vi "Mapping Countdown v10.5.1.vi"(6 "Execution Times (s)":dbl[](array[numeric]), 8 "Drive Velocity":dbl=10.0 caption="Velocity (V/s)" min=10.0 max=160.0 step=0.1 format="%.1f", 9 "Mapping Spectra Settings":T1={"Integration Time"=10.0, "Repetitions"=10, "Mapping Spectra"=TRUE} {"Repetitions" min=1 max=100 step=1; "Integration Time" min=0.5 max=6000.0 step=1.0 format="%.1f"}, 10 "Ready Steps":i32, 11 "Mapping Drive Parameters":T2={"X Start Position"=10.0, "X Stop Position"=10.0, "Y Start Position"=10.0, "Y Stop Position"=10.0, "Step Size"=10.0} {"Step Size" min=0.1 max=30.0 step=0.1 format="%.1f"; "Y Stop Position" min=0.0 max=30.0 step=0.1 format="%.1f"; "Y Start Position" min=0.0 max=30.0 step=0.1 format="%.1f"; "X Stop Position" min=0.0 max=30.0 step=0.1 format="%.1f"; "X Start Position" min=0.0 max=30.0 step=0.1 format="%.1f"}) -> (2 "Progress":i16, 3 "Time String":string)   [LabVIEW 2010]
uses:
  TypeDefs/Mapping Drive Params.ctl
  TypeDefs/Mapping Spectra Params.ctl
  <vilib>/Analysis/NI_AALBase.lvlib
panel:
  out "Step Time (s)":dbl
  out "Left Time (s)":dbl
  out "Left Steps":dbl
  out "Total Steps":dbl
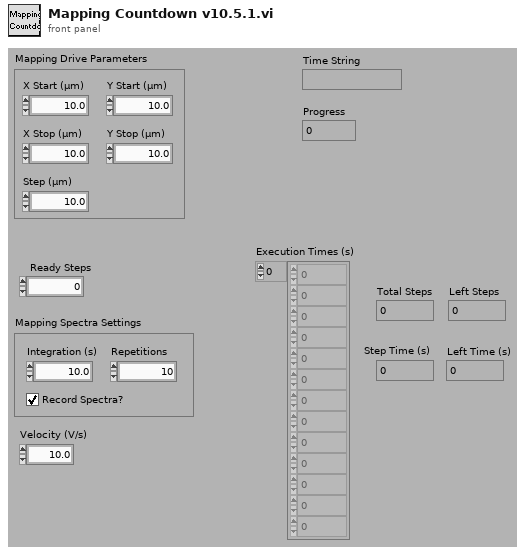
[diagram p1: front panel]
types:
  T1 = typedef "Mapping Spectra Params.ctl" = cluster{"Integration Time":dbl, "Repetitions":u16, "Mapping Spectra":bool}
  T2 = typedef "Mapping Drive Params.ctl" = cluster{"X Start Position":dbl, "X Stop Position":dbl, "Y Start Position":dbl, "Y Stop Position":dbl, "Step Size":dbl}
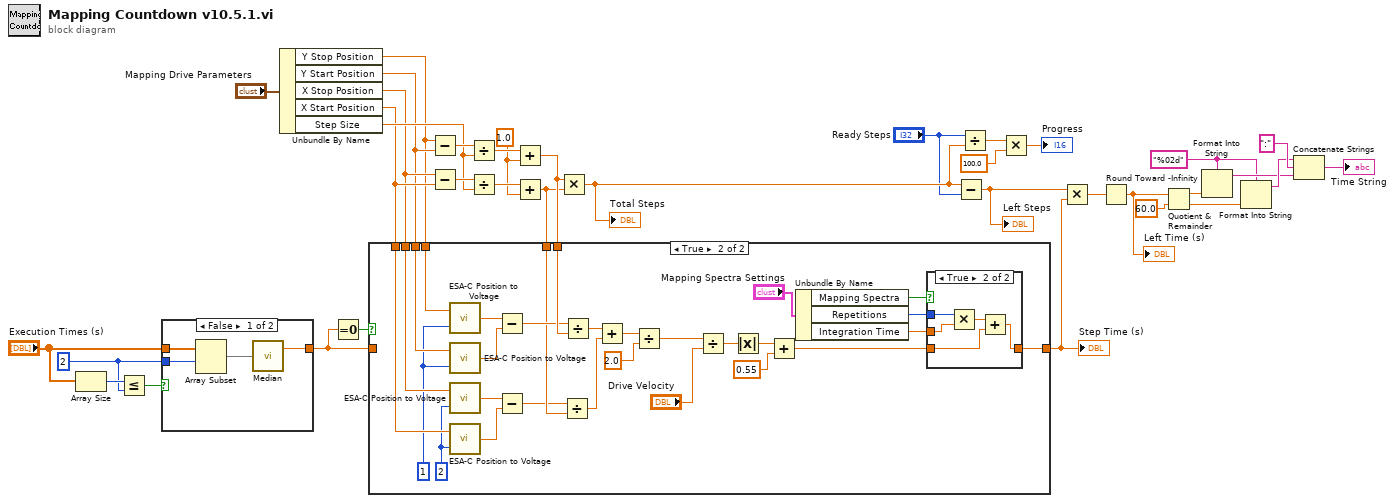
[diagram p0: block diagram]
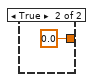
[diagram p2: hidden frame]
diagram:
  w4 = 2 ("index")
  w19 = 1.0 ("y")
  w31 = "%02d" ("Format-String")
  n1 = Array Size(array="Execution Times (s)") -> (size(s)=w7:i32)
  n2 = Less Or Equal?(x=w7, y=w4) -> (x <= y?=w6:bool)
  n3 = case shown="False" w6 {
    tunnel: "Execution Times (s)" -> [w39 _]
    tunnel: w4 -> [w38 _]
    tunnel: [w37 0.0 ("mean")] -> w3
    frame False {
      n4 = Array Subset(array=w39, index=w38) -> (w40:dbl[])  [unwired: 1 in]
      n5 = call <vilib>:"Median.vi"("X"=w40) -> ("median"=w37:dbl)  [unwired: 1 out]
    }
    frame True {
    }
  }
  n6 = Unbundle By Name("Mapping Drive Parameters") -> ("Y Stop Position"=w11:dbl, "Y Start Position"=w12:dbl, "X Stop Position"=w13:dbl, "X Start Position"=w14:dbl, "Step Size"=w15:dbl)
  n7 = Equal To 0?(x=w3) -> (x = 0?=w8:bool)
  n8 = Subtract(x=w11, y=w12) -> (x-y=w23:dbl)
  n9 = Subtract(x=w13, y=w14) -> (x-y=w22:dbl)
  n10 = Divide(x=w23, y=w15) -> (x/y=w20:dbl)
  n11 = Divide(x=w22, y=w15) -> (x/y=w21:dbl)
  n12 = Add(x=w20, y=w19) -> (x+y=w10:dbl)
  n13 = Add(x=w21, y=w19) -> (x+y=w9:dbl)
  n14 = case shown="True" w8 {
    tunnel: [w42 w66] -> w2
    tunnel: w14 -> [_ w64]
    tunnel: w13 -> [_ w63]
    tunnel: w12 -> [_ w62]
    tunnel: w11 -> [_ w61]
    tunnel: w10 -> [_ w54]
    tunnel: w9 -> [_ w52]
    tunnel: w3 -> [w42 _]
    frame False {
    }
    frame True {
      w59 = 2 ("Axis")
      w60 = 1 ("Axis")
      n15 = call "ESA-C Position to Voltage.vi"("Axis"=w60, "Position (µm)"=w61) -> ("Voltage (V)"=w58:dbl)
      n16 = call "ESA-C Position to Voltage.vi"("Axis"=w60, "Position (µm)"=w62) -> ("Voltage (V)"=w57:dbl)
      n17 = call "ESA-C Position to Voltage.vi"("Axis"=w59, "Position (µm)"=w63) -> ("Voltage (V)"=w56:dbl)
      n18 = call "ESA-C Position to Voltage.vi"("Axis"=w59, "Position (µm)"=w64) -> ("Voltage (V)"=w55:dbl)
      n19 = Subtract(x=w58, y=w57) -> (x-y=w53:dbl)
      n20 = Subtract(x=w56, y=w55) -> (x-y=w51:dbl)
      n21 = Divide(x=w51, y=w52) -> (x/y=w49:dbl)
      n22 = Divide(x=w53, y=w54) -> (x/y=w50:dbl)
      n23 = Add(x=w50, y=w49) -> (x+y=w48:dbl)
      n24 = Divide(x=w48, y=2.0) -> (x/y=w46:dbl)
      n25 = Divide(x=w46, y="Drive Velocity") -> (x/y=w44:dbl)
      n26 = Absolute Value(x=w44) -> (abs(x)=w43:dbl)
      n27 = Add(x=w43, y=0.55) -> (x+y=w65:dbl)
      n28 = Unbundle By Name("Mapping Spectra Settings") -> ("Mapping Spectra"=w69:bool, "Repetitions"=w68:u16, "Integration Time"=w67:dbl)
      n29 = case shown="True" w69 {
        tunnel: w68 -> [_ w77]
        tunnel: w67 -> [_ w76]
        tunnel: w65 -> [w72 w74]
        tunnel: [w72 w73] -> w66
        frame False {
        }
        frame True {
          n30 = Multiply(x=w77, y=w76) -> (x*y=w75:dbl)
          n31 = Add(x=w75, y=w74) -> (x+y=w73:dbl)
        }
      }
    }
  }
  "Step Time (s)" <- w2
  n32 = Multiply(x=w10, y=w9) -> (x*y=w18:dbl)
  "Total Steps" <- w18
  n33 = Subtract(x=w18, y="Ready Steps") -> (x-y=w17:dbl)
  "Left Steps" <- w17
  n34 = Divide(x="Ready Steps", y=w18) -> (x/y=w16:dbl)
  n35 = Multiply(x=w16, y=100.0) -> (x*y=→"Progress":dbl)
  n36 = Multiply(x=w17, y=w2) -> (x*y=w25:dbl)
  n37 = Round Toward -Infinity(1:w25) -> (0:w28:dbl)
  "Left Time (s)" <- w28
  n38 = Quotient & Remainder(x=w28, y=60.0) -> (x-y*floor(x/y)=w30:dbl, floor(x/y)=w29:dbl)
  n39 = Format Into String(format string=w31, w30) -> (resulting string=w32:string)  [unwired: 2 in, 1 out]
  n40 = Format Into String(format string=w31, w29) -> (resulting string=w33:string)  [unwired: 2 in, 1 out]
  n41 = Concatenate Strings(w33, ":" ("String"), w32) -> (→"Time String":string)
